vi "Run_Init Core.vi"(0 "functionbase in":refnum<class "functionbase.lvclass">, 11 "error in (no error)":errorcluster) -> (4 "functionbase out":refnum<class "functionbase.lvclass">, 15 "error out":errorcluster)   [LabVIEW 2016, in "functionbase.lvclass"]
uses:
  functionbase.lvclass
  functionbase.lvclass/functionbase.ctl
  properties/Read RT Variables.vi
  variables/RT Variables/RT Variables.lvclass
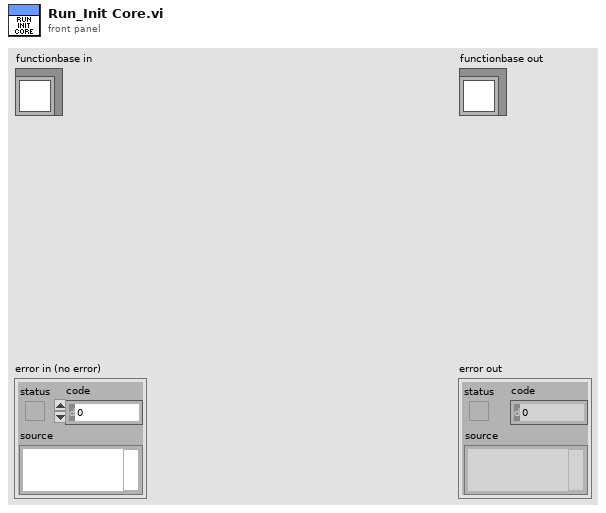
[diagram p1: front panel]
types:
  T1 = typedef "Datatype.ctl" = enum16{"Null", "Numeric", "String", "Bool", "Numeric 1D", "String 1D", "Bool 1D", "Numeric 2D", "String 2D", "Bool 2D", "Variant"}
  T2 = typedef "Valuetype.ctl" = enum16{"Value", "Variable", "Function"}
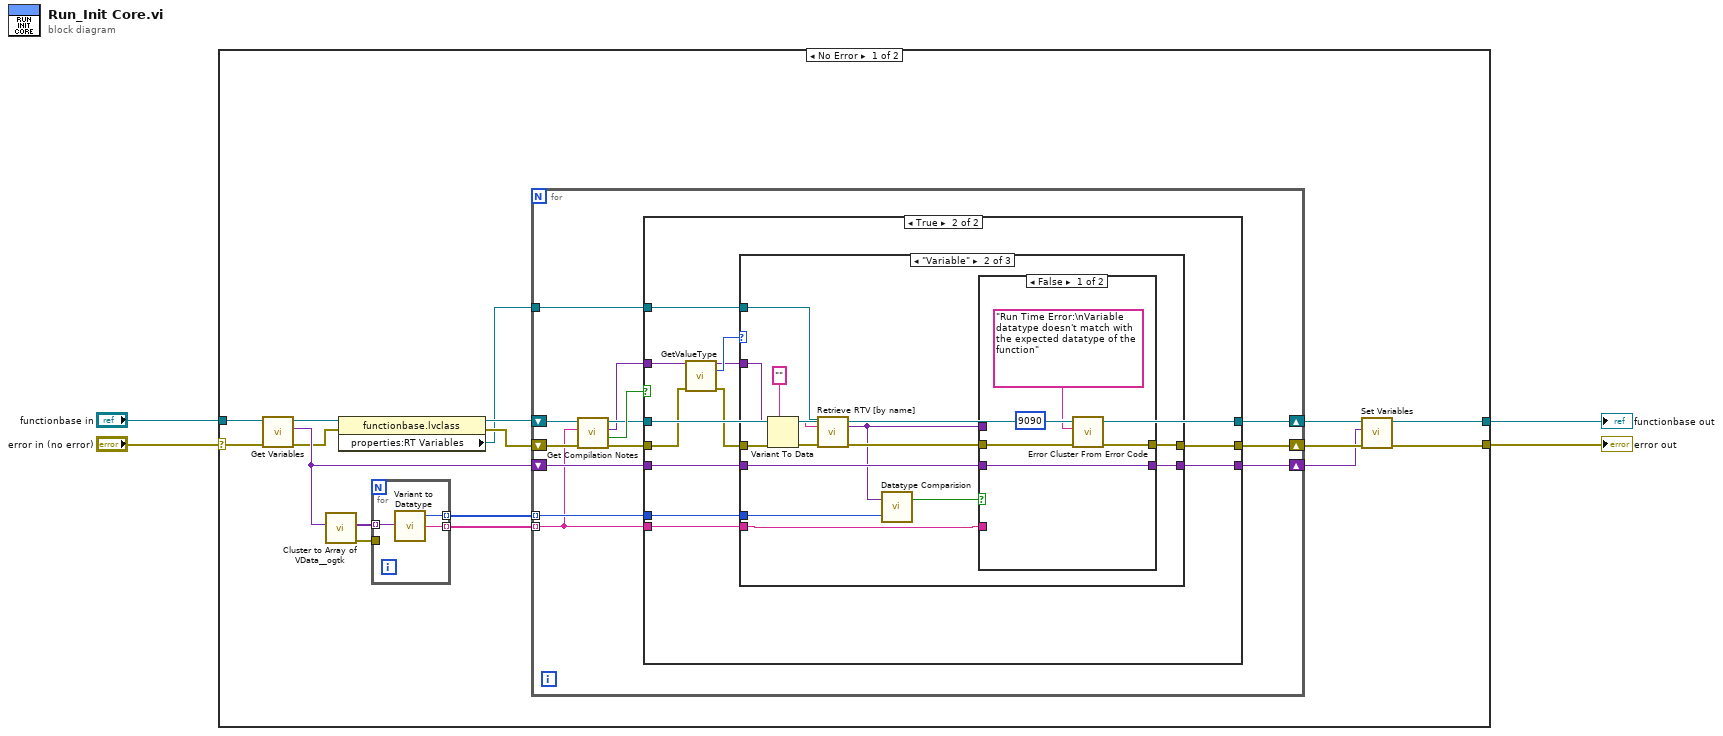
[diagram p0: block diagram]
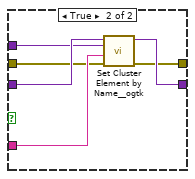
[diagram p4: hidden frame]
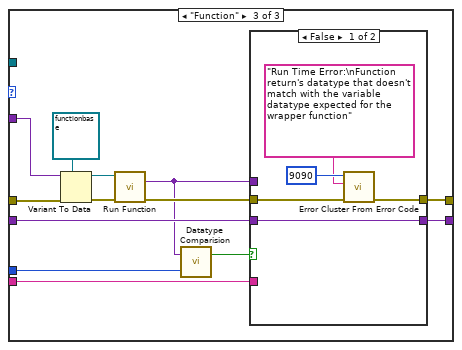
[diagram p5: hidden frame]
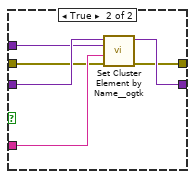
[diagram p6: hidden frame]
diagram:
  n1 = case shown="No Error" "error in (no error)" {
    selector: "error in (no error)" -> [w20 w105]
    tunnel: [w12 w105] -> w3
    tunnel: [w11 w104] -> w1
    tunnel: "functionbase in" -> [w19 w104]
    frame No Error {
      n2 = call-dynamic "Get Variables.vi"("error in (no error)"=w20, "functionbase in"=w19) -> ("error out"=w7:errorcluster, "Variables"=w16:variant, "functionbase out"=w9:refnum<class "functionbase.lvclass">)  [unwired: 7 in]
      n3 = call <userlib>:"Cluster to Array of VData__ogtk.vi"("Cluster"=w16) -> ("error out"=w18:errorcluster, "Array of VData"=w21:variant[])  [unwired: 9 in]
      n4 = property class="functionbase.lvclass"(reference=w9, error in=w7) -> (reference out=w8:refnum<class "functionbase.lvclass">, error out=w6:errorcluster, "properties:RT Variables"=w5:refnum<class "RT Variables.lvclass">)
      n5 = for {
        tunnel: w21 -> [w103] mode=indexing
        tunnel: [w102] -> w10 mode=indexing
        tunnel: [w101] -> w17 mode=indexing
        tunnel: w18 -> [_]
        n6 = call "Variant to Datatype.vi"("Variant"=w103) -> ("Name"=w101:string, "Datatype"=w102:T1)  [unwired: 2 in, 1 out]
      }
      n7 = for {
        shift-right: [w25] -> w15
        shift-left: w8 -> [w33]
        tunnel: w17 -> [w23] mode=indexing
        shift-right: [w31] -> w13
        shift-left: w16 -> [w32]
        shift-right: [w26] -> w14
        shift-left: w6 -> [w34]
        tunnel: w10 -> [w24] mode=indexing
        tunnel: w5 -> [w22]
        n8 = call "Get Compilation Notes.vi"("error in (no error)"=w34, "note key"=w23, "functionbase in"=w33) -> ("error out"=w28:errorcluster, "Found?"=w30:bool, "Notes"=w27:variant, "functionbase out"=w29:refnum<class "functionbase.lvclass">)  [unwired: 5 in]
        n9 = case shown="True" w30 {
          tunnel: w32 -> [w35 w43]
          tunnel: [w35 w44] -> w31
          tunnel: w29 -> [w37 w49]
          tunnel: w28 -> [w36 w47]
          tunnel: w27 -> [_ w48]
          tunnel: [w36 w42] -> w26
          tunnel: [w37 w49] -> w25
          tunnel: w24 -> [_ w40]
          tunnel: w23 -> [_ w39]
          tunnel: w22 -> [_ w38]
          frame False {
          }
          frame True {
            n10 = call "GetValueType.vi"("variant"=w48, "error in"=w47) -> ("variant out"=w45:variant, "Value Type"=w46:T2, "error out"=w41:errorcluster)  [unwired: 11 in]
            n11 = case shown="\"Variable\"" w46 {
              tunnel: w45 -> [_ w64 w88]
              tunnel: [w51 w60 w83] -> w44
              tunnel: w43 -> [w51 w61 w84]
              tunnel: [w50 w59 w80] -> w42
              tunnel: w41 -> [w50 w65 w89]
              tunnel: w40 -> [_ w56 w78]
              tunnel: w39 -> [_ w57 w82]
              tunnel: w38 -> [_ w53 _]
              frame "Value", Default {
              }
              frame "Variable" {
                n12 = Variant To Data(error in=w65, type="", Variant=w64) -> (data=w54:string, error out=w62:errorcluster)
                n13 = call-dynamic "Retrieve RTV [by name].vi"("RT Variables in"=w53, "RTV name"=w54, "error in (no error)"=w62) -> ("Data"=w52:variant, "error out"=w58:errorcluster)  [unwired: 8 in, 3 out]
                n14 = call "Datatype Comparision.vi"("Required Datatype"=w56, "Data"=w52) -> ("Equal?"=w55:bool)  [unwired: 1 in]
                n15 = case shown="False" w55 {
                  tunnel: w61 -> [w70 w76]
                  tunnel: [w70 w75] -> w60
                  tunnel: w52 -> [_ w74]
                  tunnel: w57 -> [_ w73]
                  tunnel: w58 -> [w69 w72]
                  tunnel: [w68 w71] -> w59
                  frame False {
                    n16 = call <vilib>:"Error Cluster From Error Code.vi"("error in (no error)"=w69, "error message (\"\")"="Run Time Error:\nVariable datatype doesn't match with the expected datatype of the function" ("error message (\"\")"), "error code (0)"=9090) -> ("error out"=w68:errorcluster)  [unwired: 6 in]
                  }
                  frame True {
                    n17 = call <userlib>:"Set Cluster Element by Name__ogtk.vi"("error in (no error)"=w72, "Element Name (\"\": New Element Data Name)"=w73, "New Element Value"=w74, "Cluster"=w76) -> ("error out"=w71:errorcluster, "VCluster out"=w75:variant)  [unwired: 5 in, 1 out]
                  }
                }
              }
              frame "Function" {
                n18 = Variant To Data(error in=w89, type=refnum<class "functionbase.lvclass"> refnum ("functionbase.lvclass"), Variant=w88) -> (data=w86:refnum<class "functionbase.lvclass">, error out=w85:errorcluster)
                n19 = call-dynamic "Run Function.vi"("functionbase in"=w86, "error in (no error)"=w85) -> ("Return"=w79:variant, "error out"=w81:errorcluster)  [unwired: 11 in, 1 out]
                n20 = call "Datatype Comparision.vi"("Required Datatype"=w78, "Data"=w79) -> ("Equal?"=w77:bool)  [unwired: 1 in]
                n21 = case shown="False" w77 {
                  tunnel: w84 -> [w94 w100]
                  tunnel: [w94 w99] -> w83
                  tunnel: w79 -> [_ w98]
                  tunnel: w82 -> [_ w97]
                  tunnel: w81 -> [w93 w96]
                  tunnel: [w92 w95] -> w80
                  frame False {
                    n22 = call <vilib>:"Error Cluster From Error Code.vi"("error in (no error)"=w93, "error message (\"\")"="Run Time Error:\nFunction return's datatype that doesn't match with the variable datatype expected for the wrapper function" ("error message (\"\")"), "error code (0)"=9090) -> ("error out"=w92:errorcluster)  [unwired: 6 in]
                  }
                  frame True {
                    n23 = call <userlib>:"Set Cluster Element by Name__ogtk.vi"("error in (no error)"=w96, "Element Name (\"\": New Element Data Name)"=w97, "New Element Value"=w98, "Cluster"=w100) -> ("error out"=w95:errorcluster, "VCluster out"=w99:variant)  [unwired: 5 in, 1 out]
                  }
                }
              }
            }
          }
        }
      }
      n24 = call-dynamic "Set Variables.vi"("error in (no error)"=w14, "Variables"=w13, "functionbase in"=w15) -> ("error out"=w12:errorcluster, "functionbase out"=w11:refnum<class "functionbase.lvclass">)  [unwired: 7 in]
    }
    frame Error {
    }
  }
  "error out" <- w3
  "functionbase out" <- w1
